vi "ToolScan單步驟測試.vi"() -> ()   [LabVIEW 2019]
uses:
  Ctrl/ProjectStepSelect.ctl
panel:
  out "error out":errorcluster
  in  "error in (no error)":errorcluster
  out "read string 6":string
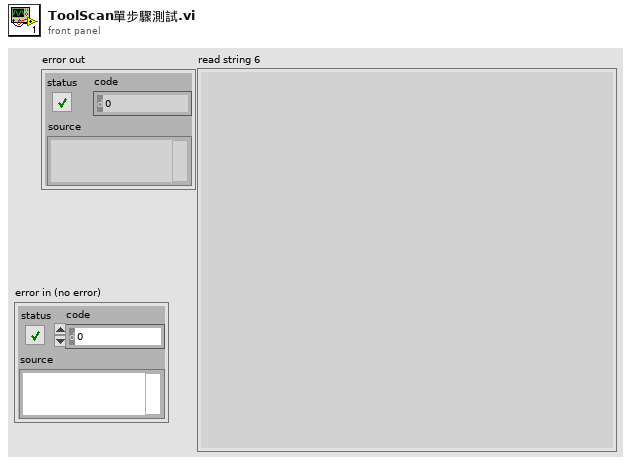
[diagram p1: front panel]
types:
  T1 = typedef "ProjectStepSelect.ctl" = enum16{"ProjectName", "Name", "Initial", "Reset", "Format", "Program1", "Program2", "Scan", "Finish", "MToolWork", "DataCheck", "DataSave", "OutputPLC", "WaitInputS1", "WaitInputOff"}
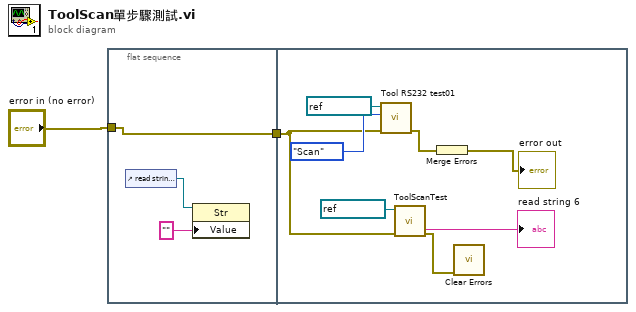
[diagram p0: block diagram]
diagram:
  n1 = flat-sequence {
    tunnel: "error in (no error)" -> [w3]
    tunnel: [w3] -> w1
    tunnel: w1 -> [w9]
    frame #0 {
      n2 = control-ref of="read string 6"() -> (w5:refnum<vi>)
      n3 = property class="Str"(reference=w5, "Value"="") -> ()  [unwired: 1 in, 2 out]
    }
    frame #1 {
      n4 = call "Tool RS232 test01.vi"("error in (no error)"=w9, "select step"=ProjectStepSelect."Scan", "VISA resource name"=refnum<visa-resource-name> "COM3") -> ("error out"=w8:errorcluster)  [unwired: 8 in]
      n5 = call "ToolScanTest.vi"("error in (no error)"=w9, "VISA resource name"=refnum<visa-resource-name> "COM5") -> ("error out"=w6:errorcluster, "read string 6"=→"read string 6":string)  [unwired: 5 in, 3 out]
      n6 = Merge Errors(w8) -> (→"error out":errorcluster)
      n7 = call <vilib>:"Clear Errors.vi"("error in (no error)"=w6) -> ()  [unwired: 5 in, 2 out]
    }
  }
